vi "Hadamard Matrix (DBL).vi"(11 "matrix size":i32) -> (0 "error":i32, 3 "Hadamard Matrix":T1)   [LabVIEW 2024, in "NI_AALPro.lvlib"]
uses:
  NI_AALPro.lvlib
  RealMatrix.ctl
  NI_Matrix.lvlib
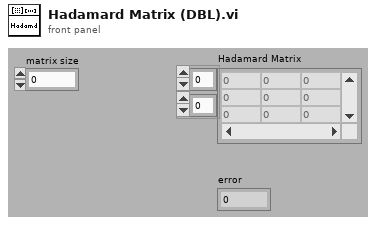
[diagram p1: front panel]
types:
  T1 = typedef "NI_Matrix.lvlib/RealMatrix.ctl" = dbl[][]
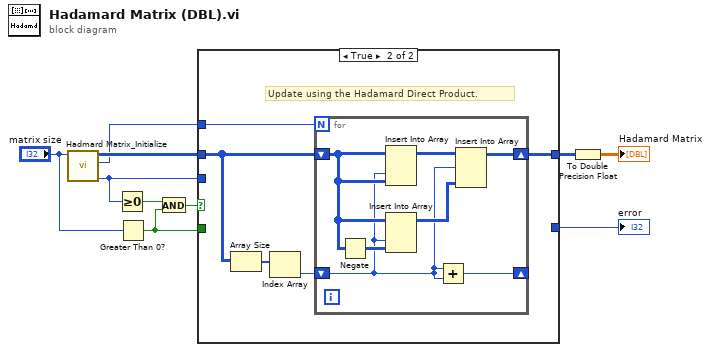
[diagram p0: block diagram]
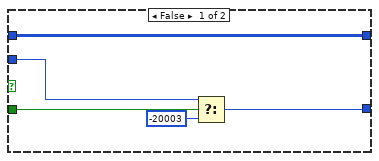
[diagram p2: hidden frame]
diagram:
  n1 = call "Hadmard Matrix_Initialize.vi"("matrix size"="matrix size") -> ("error"=w2:i32, "k [m*2^k=n]"=w9:i32, "Initial Hadamard Matrix"=w10:i8[][])  [unwired: 8 out]
  n2 = Greater Or Equal To 0?(x=w2) -> (x >= 0?=w5:bool)
  n3 = Greater Than 0?(x="matrix size") -> (x > 0?=w3:bool)
  n4 = And(x=w5, y=w3) -> (x .and. y?=w4:bool)
  n5 = case shown="True" w4 {
    tunnel: w10 -> [w15 w18]
    tunnel: [w15 w20] -> w8
    tunnel: w9 -> [_ w19]
    tunnel: w3 -> [w14 _]
    tunnel: w2 -> [w12 _]
    tunnel: [w11 _] -> w1
    frame False {
      n6 = Select(t=w12, s=w14, f=-20003) -> (s? t:f=w11:i32)
    }
    frame True {
      # "Update using the Hadamard Direct Product."
      n7 = Array Size(array=w18) -> (size(s)=w16:i32[])
      n8 = Index Array(array=w16) -> (element=w17:i32)  [unwired: 1 in]
      n9 = for {
        N: w19 -> [_]
        shift-right: [w23] -> w20
        shift-left: w18 -> [w24]
        shift-right: [w22] -> _
        shift-left: w17 -> [w21]
        n10 = Negate(x=w24) -> (-x=w26:i8[][])
        n11 = Insert Into Array(array=w24, index (col)=w21, new element=w24) -> (w27:i8[][])  [unwired: 1 in]
        n12 = Insert Into Array(array=w24, index (col)=w21, new element=w26) -> (w25:i8[][])  [unwired: 1 in]
        n13 = Add(x=w21, y=w21) -> (x+y=w22:i32)
        n14 = Insert Into Array(array=w27, index (row)=w21, new element=w25) -> (w23:i8[][])  [unwired: 1 in]
      }
    }
  }
  "error" <- w1
  n15 = To Double Precision Float(number=w8) -> (double precision float=→"Hadamard Matrix":dbl[][])
